vi "Code128(B)Build-Zxing.vi"(2 "ScaleY":u8=4, 3 "ScaleX":u8=1, 5 "Text":string="ZY201801") -> (1 "out Array":bool[][](array[boolean]))   [LabVIEW 2018]
uses:
  zxing.dll
panel:
  out "大小":i32[](array[numeric])
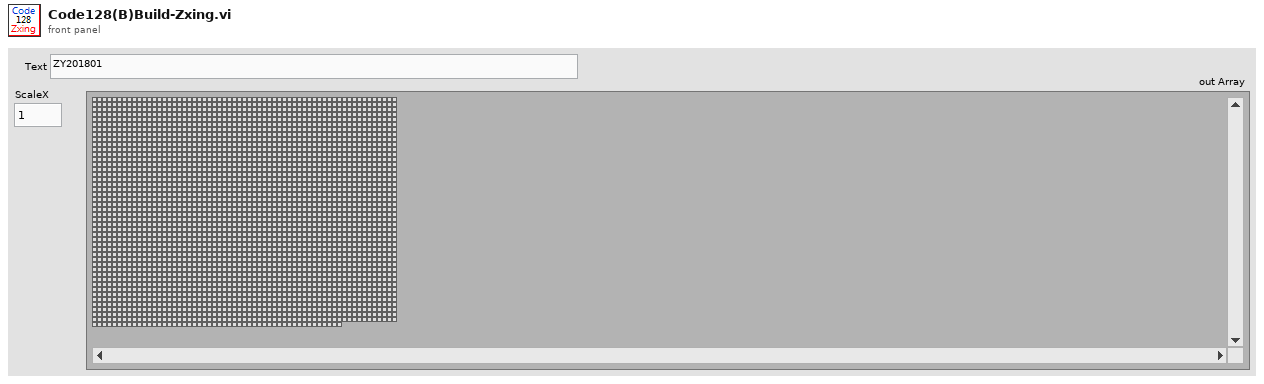
[diagram p1: front panel]
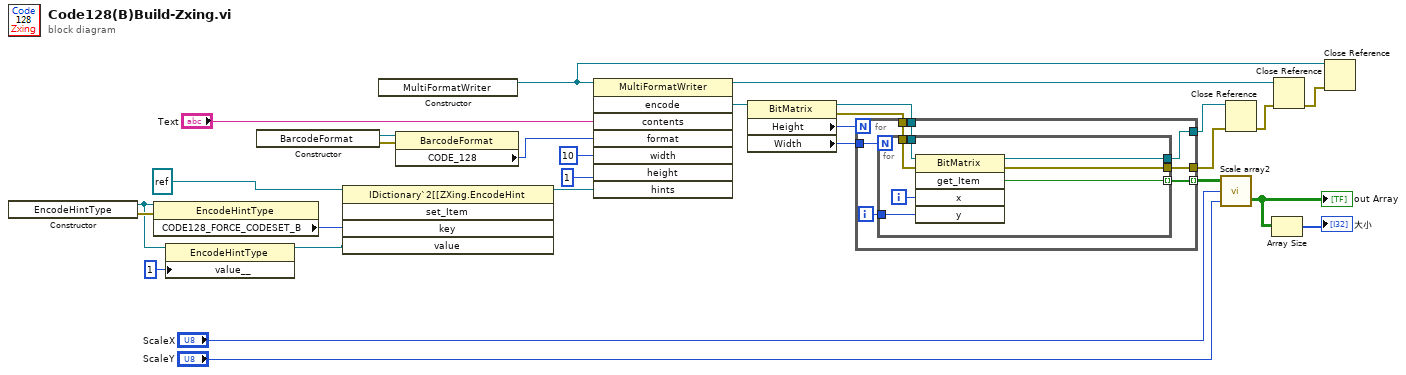
[diagram p0: block diagram]
diagram:
  n1 = constructor class="EncodeHintType"() -> (reference out=w2:refnum<k24>, error out=w13:errorcluster)  [unwired: 3 in, 1 out]
  n2 = property class="EncodeHintType"(reference=w2, error in=w13) -> ("CODE128_FORCE_CODESET_B"=w6:i32)  [unwired: 2 out]
  n3 = property class="EncodeHintType"(reference=w2, "value__"=1) -> (reference out=w3:refnum<k24>)  [unwired: 1 in, 1 out]
  n4 = constructor class="BarcodeFormat"() -> (reference out=w9:refnum<k24>, error out=w10:errorcluster)  [unwired: 3 in, 1 out]
  n5 = invoke class="IDictionary`2[[ZXing.EncodeHint" method="set_Item"(reference=refnum<k24> refnum ("引用"), "key"=w6, "value"=w3) -> (reference out=w7:refnum<k24>)  [unwired: 2 in, 4 out]
  n6 = constructor class="MultiFormatWriter"() -> (reference out=w4:refnum<k24>)  [unwired: 3 in, 2 out]
  n7 = property class="BarcodeFormat"(reference=w9, error in=w10) -> ("CODE_128"=w8:i32)  [unwired: 2 out]
  n8 = invoke class="MultiFormatWriter" method="encode"(reference=w4, "contents"="Text", "format"=w8, "width"=10, "height"=1, "hints"=w7) -> (reference out=w12:refnum<k24>, "encode"=w16:refnum<k24>)  [unwired: 2 in, 6 out]
  n9 = property class="BitMatrix"(reference=w16) -> (reference out=w26:refnum<k24>, error out=w25:errorcluster, "Height"=w29:i32, "Width"=w28:i32)  [unwired: 1 in]
  n10 = for {
    N: w29 -> [_]
    tunnel: w28 -> [w36]
    tunnel: [w34] -> w21 mode=indexing
    tunnel: [w33] -> w23
    tunnel: [w32] -> w24
    tunnel: w26 -> [w31]
    tunnel: w25 -> [w30]
    i -> [w35]
    n11 = for {
      N: w36 -> [_]
      tunnel: w35 -> [w42]
      tunnel: [w37] -> w34 mode=indexing
      tunnel: [w41] -> w33
      tunnel: [w38] -> w32
      tunnel: w31 -> [w40]
      tunnel: w30 -> [w39]
      i -> [w43]
      n12 = invoke class="BitMatrix" method="get_Item"(reference=w40, error in=w39, "x"=w43, "y"=w42) -> (reference out=w41:refnum<k24>, error out=w38:errorcluster, "get_Item"=w37:bool)  [unwired: 1 in, 2 out]
    }
  }
  n13 = call "Scale array2.vi"("ScaleY"="ScaleY", "ScaleX"="ScaleX", "in Array"=w21) -> ("out Array"=w18:bool[][])  [unwired: 2 in]
  "out Array" <- w18
  n14 = Close Reference(reference=w23, error in (no error)=w24) -> (error out=w27:errorcluster)
  n15 = Array Size(array=w18) -> (size(s)=→"大小":i32[])
  n16 = Close Reference(reference=w12, error in (no error)=w27) -> (error out=w22:errorcluster)
  n17 = Close Reference(reference=w4, error in (no error)=w22) -> ()  [unwired: 1 out]
